vi "test boolean strings.vi"() -> ()   [LabVIEW 2017]
uses:
  c3e610f3-1f6a-439d-9ae6-4bf36613db9f.vi
  addons/API-String-Arugments-Support/_Support/Convert API String Arguments to Data(variant).vi
  addons/API-String-Arugments-Support/API String Arguments Support.lvlib
panel:
  out "True Boolean Strings":string[](array[string])
  out "error":errorcluster
  out "Data":bool
  in  "String":string
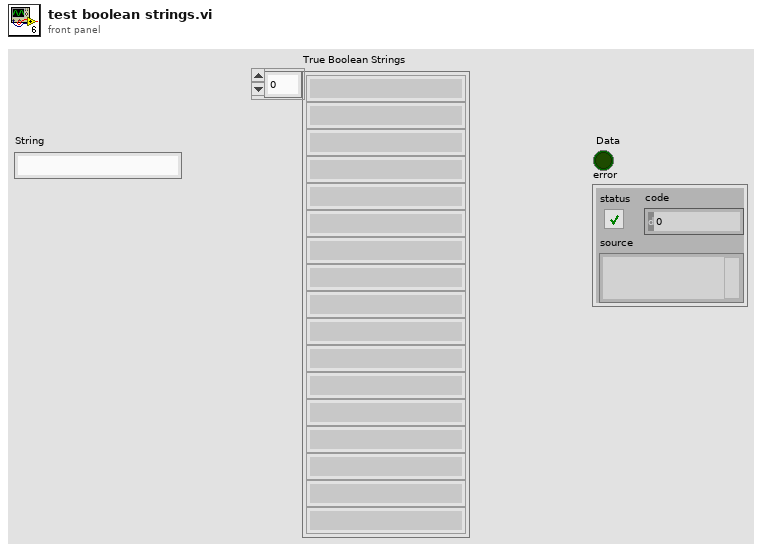
[diagram p1: front panel]
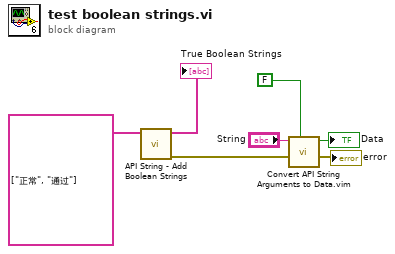
[diagram p0: block diagram]
diagram:
  n1 = call "API String - Add Boolean Strings.vi"("Customer True Boolean Strings"=string[] ["正常", "通过"]) -> ("Error out"=w7:errorcluster, "True Boolean Strings"=→"True Boolean Strings":string[])  [unwired: 8 in, 1 out]
  n2 = call "Convert API String Arguments to Data.vim"("Type"=FALSE, "error in (no error)"=w7, "String"="String") -> ("error"=→"error":errorcluster, "Data"=→"Data":bool)  [unwired: 5 in]
